vi "动态时间的规整.vi"(1 "参考模板特征":dbl[][](array[numeric]) format="%.2f", 2 "²âÊÔÄ£°åÌØÕ÷Å":dbl[][](array[numeric]) format="%.2f") -> (0 "距离":dbl)   [LabVIEW 2018]
panel:
  out "错误输出":errorcluster
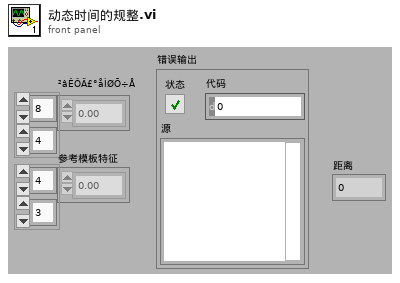
[diagram p1: front panel]
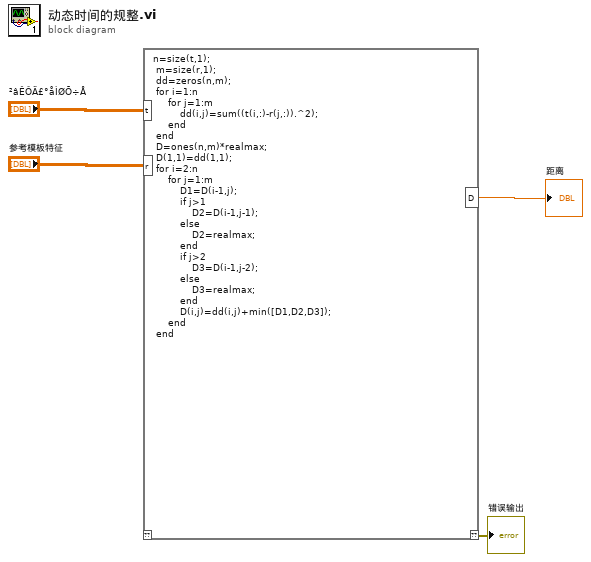
[diagram p0: block diagram]
diagram:
  n1 = script code="n=size(t,1);\n m=size(r,1);\n dd=zeros(n,m);\n for i=1:n\n     for j=1:m\n         dd(i,j)=sum((t(i,:)-r(j,:)).^2);\n     end\n end\n D=ones(n,m)*realmax;\n D(1,1)=dd(1,1);\n for i=2:n\n     for j=1:m\n         D1=D(i-1,j);\n         if j>1\n             D2=D(i-1,j-1);\n         else\n             D2=realmax;\n         end\n         if j>2\n             D3=D(i-1,j-2);\n         else\n             D3=realmax;\n         end\n         D(i,j)=dd(i,j)+min([D1,D2,D3]);\n     end\n end"("t"="²âÊÔÄ£°åÌØÕ÷Å", "r"="参考模板特征") -> ("??"=→"错误输出":errorcluster, "D"=→"距离":dbl)  [unwired: 1 in]
